vi "Cn.vi"(9 "l":dbl, 10 "beta":dbl, 11 "alpha":dbl) -> (3 "Array":dbl[](array[numeric]))   [LabVIEW 2011]
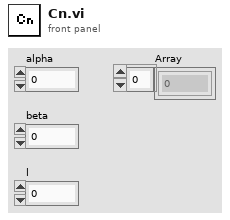
[diagram p1: front panel]
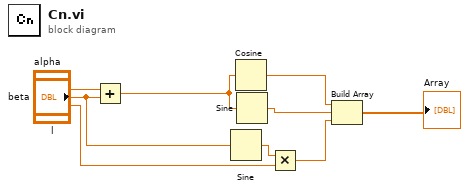
[diagram p0: block diagram]
diagram:
  n1 = Add(x="alpha", y="beta") -> (x+y=w2:dbl)
  n2 = Sine(x="beta") -> (sin(x)=w4:dbl)
  n3 = Cosine(x=w2) -> (cos(x)=w6:dbl)
  n4 = Sine(x=w2) -> (sin(x)=w7:dbl)
  n5 = Multiply(x=w4, y="l") -> (x*y=w8:dbl)
  n6 = Build Array(w6, w7, w8) -> (→"Array":dbl[])
